vi "Create Report.vi"(7 "Print Report?":bool=TRUE, 8 "error in":errorcluster, 9 "Test Results":string[][](array[string]), 10 "Test Info":string[][](array[string])) -> (0 "error out":errorcluster)   [LabVIEW 2010]
uses:
  <vilib>/Utility/NIReport.llb/NI_report.lvclass
  <vilib>/Utility/NIReport.llb/Append Report Text (str wrap).vi
  <vilib>/Utility/NIReport.llb/Append Text Table to Report (wrap).vi
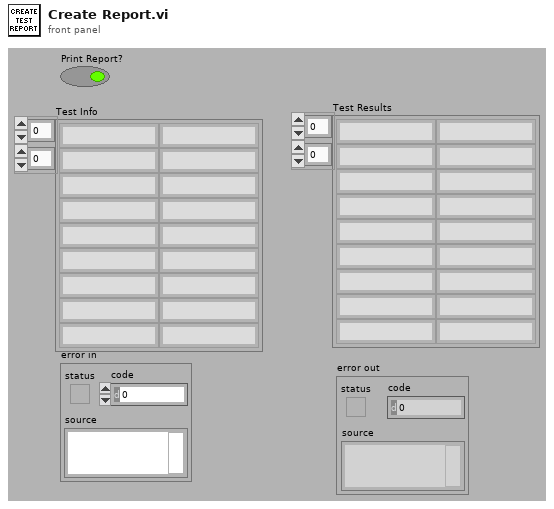
[diagram p1: front panel]
types:
  T1 = cluster{"Charset (-1)":i16, "Weight (-1)":i16, "Name":string, "Size":string}
  T2 = enum16{"Standard Report", "HTML", "Word", "Excel"}
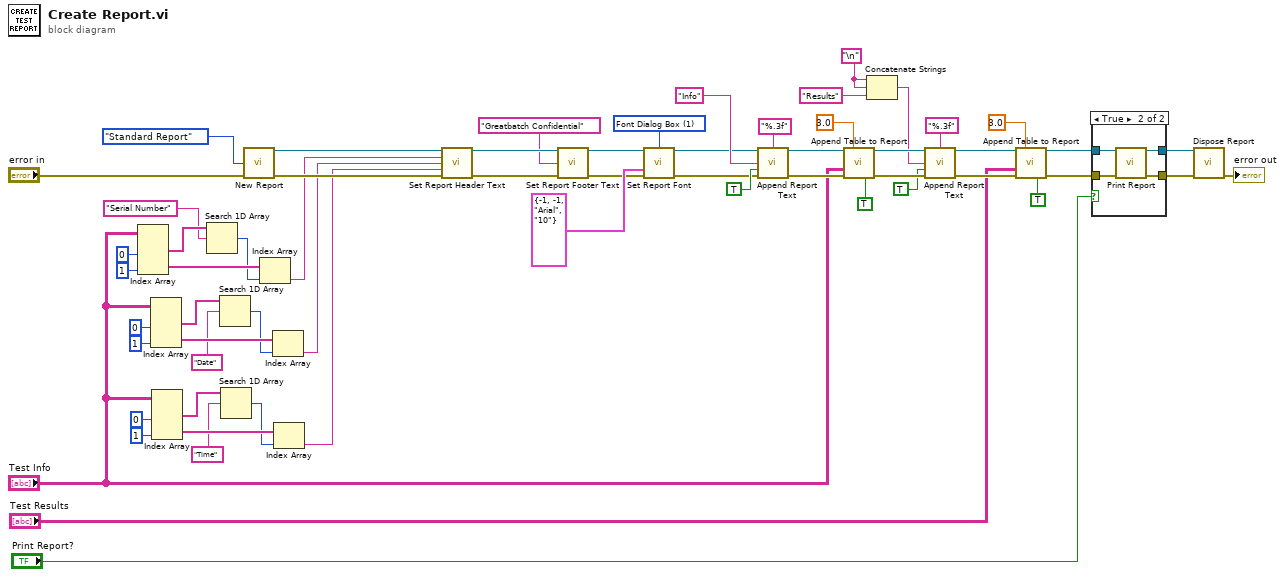
[diagram p0: block diagram]
diagram:
  w3 = "\n"
  w40 = u16 1 items=["VI Inputs", "Font Dialog Box"] ("font settings source")
  n1 = Index Array(array="Test Info", index (col) #1=0 ("disabled index (col)"), index (col) #2=1 ("index (col)")) -> (element #1=w38:string[], element #2=w36:string[])  [unwired: 2 in]
  n2 = Index Array(array="Test Info", index (col) #1=0 ("disabled index (col)"), index (col) #2=1 ("index (col)")) -> (element #1=w20:string[], element #2=w18:string[])  [unwired: 2 in]
  n3 = Index Array(array="Test Info", index (col) #1=0 ("disabled index (col)"), index (col) #2=1 ("index (col)")) -> (element #1=w14:string[], element #2=w12:string[])  [unwired: 2 in]
  n4 = Search 1D Array(1D array=w38, element="Serial Number") -> (index of element=w35:i32)  [unwired: 1 in]
  n5 = Search 1D Array(1D array=w20, element="Date") -> (index of element=w17:i32)  [unwired: 1 in]
  n6 = Search 1D Array(1D array=w14, element="Time") -> (index of element=w11:i32)  [unwired: 1 in]
  n7 = call <vilib>:"New Report.vi"("report type"=T2."Standard Report", "error in (no error)"="error in") -> ("report out"=w23:refnum<class "NI_report.lvclass">, "error out"=w22:errorcluster)  [unwired: 12 in]
  n8 = Index Array(array=w36, index=w35) -> (element=w6:string)
  n9 = Index Array(array=w18, index=w17) -> (element=w8:string)
  n10 = Index Array(array=w12, index=w11) -> (element=w7:string)
  n11 = call-dynamic "Set Report Header Text.vi"("report in"=w23, "left header text"=w6, "center header text"=w8, "right header text"=w7, "error in (no error)"=w22) -> ("report out"=w33:refnum<class "NI_report.lvclass">, "error out"=w31:errorcluster)  [unwired: 9 in]
  n12 = call-dynamic "Set Report Footer Text.vi"("report in"=w33, "center footer text"="Greatbatch Confidential", "error in (no error)"=w31) -> ("report out"=w32:refnum<class "NI_report.lvclass">, "error out"=w30:errorcluster)  [unwired: 11 in]
  n13 = call-dynamic "Set Report Font.vi"("report in"=w32, "font settings source"=w40, "font settings"=T1 {"Charset (-1)"=-1, "Weight (-1)"=-1, "Name"="Arial", "Size"="10"}, "error in (no error)"=w30) -> ("report out"=w43:refnum<class "NI_report.lvclass">, "error out"=w42:errorcluster)  [unwired: 9 in, 1 out]
  n14 = call-poly <vilib>:"Append Report Text.vi"("report in"=w43, "format string (%.3f)"="%.3f", "text"="Info", "append on new line? (F)"=TRUE, "error in (no error)"=w42) -> ("report out"=w44:refnum<class "NI_report.lvclass">, "error out"=w45:errorcluster)  [unwired: 7 in, 2 out]
  n15 = call-poly <vilib>:"Append Table to Report.vi"("report in"=w44, "column width (1)"=3.0, "text data"="Test Info", "error in (no error)"=w45, "show grid lines"=TRUE) -> ("report out"=w56:refnum<class "NI_report.lvclass">, "error out"=w55:errorcluster)  [unwired: 7 in, 2 out]
  n16 = Concatenate Strings(w3, w3, "Results") -> (w5:string)
  n17 = call-poly <vilib>:"Append Report Text.vi"("report in"=w56, "format string (%.3f)"="%.3f", "text"=w5, "append on new line? (F)"=TRUE, "error in (no error)"=w55) -> ("report out"=w50:refnum<class "NI_report.lvclass">, "error out"=w49:errorcluster)  [unwired: 7 in, 2 out]
  n18 = call-poly <vilib>:"Append Table to Report.vi"("report in"=w50, "column width (1)"=3.0, "text data"="Test Results", "error in (no error)"=w49, "show grid lines"=TRUE) -> ("report out"=w1:refnum<class "NI_report.lvclass">, "error out"=w2:errorcluster)  [unwired: 7 in, 2 out]
  n19 = case shown="True" "Print Report?" {
    tunnel: [w61 w65] -> w27
    tunnel: [w62 w66] -> w28
    tunnel: w2 -> [w61 w64]
    tunnel: w1 -> [w62 w63]
    frame False {
    }
    frame True {
      n20 = call-dynamic "Print Report.vi"("report in"=w63, "error in (no error)"=w64) -> ("report out"=w66:refnum<class "NI_report.lvclass">, "error out"=w65:errorcluster)  [unwired: 12 in]
    }
  }
  n21 = call-dynamic "Dispose Report.vi"("report in"=w28, "error in (no error)"=w27) -> ("error out"=→"error out":errorcluster)  [unwired: 13 in]
